vi "Output.vi"() -> ()   [LabVIEW 2011]
uses:
  Globals/Global IO.vi
panel:
  in  "DO":bool[](array[boolean])
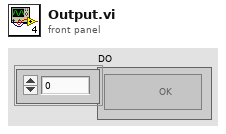
[diagram p1: front panel]
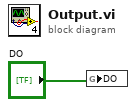
[diagram p0: block diagram]
diagram:
  n1 = global write "Global IO.vi" "DO"("DO") -> ()
